vi "AWG Stop Pulses.vi"(8 "error in (no error)":errorcluster, 11 "awg session in":T1) -> (0 "error out":errorcluster, 3 "awg session out":T1)   [LabVIEW 2013, in "AWG.lvlib"]
doc: "AWG wrapper: Stops generation of pulses at output. At least for 33120 model this should be called first after initialization to stop standard waveform mode, i.e. to stop output."
uses:
  AWG.lvlib
  AWG Session.ctl
  AWG Type.ctl
  Agilent 33XXX Series/Agilent 33XXX Series.lvlib
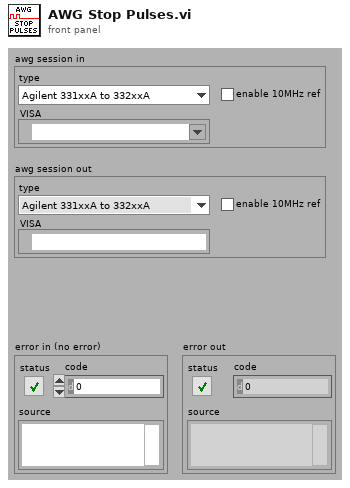
[diagram p1: front panel]
types:
  T1 = typedef "AWG.lvlib/AWG Session.ctl" = cluster{"type":T2, "VISA":refnum<visa-resource-name>, "enable 10MHz ref":bool}
  T2 = typedef "AWG.lvlib/AWG Type.ctl" = enum16{"Agilent 331xxA to 332xxA", "Agilent 335xxA to 336xxA", "dummy"}
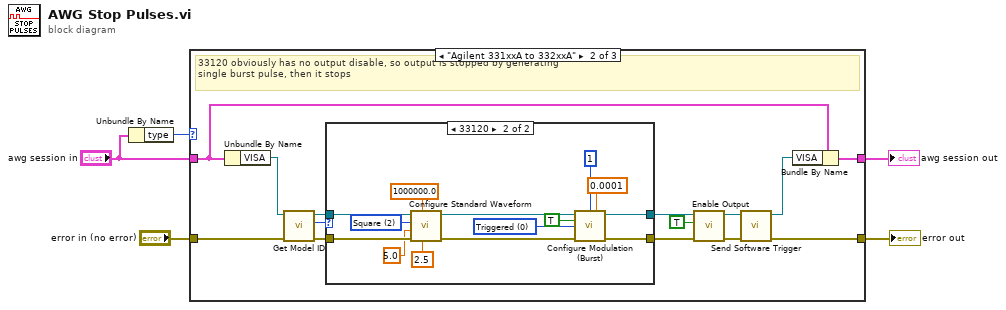
[diagram p0: block diagram]
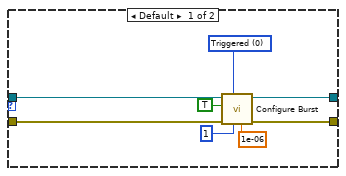
[diagram p3: hidden frame]
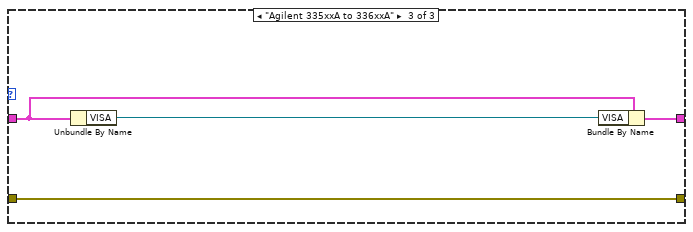
[diagram p4: hidden frame]
diagram:
  n1 = Unbundle By Name("awg session in") -> ("type"=w5:T2)
  n2 = case shown="\"Agilent 331xxA to 332xxA\"" w5 {
    tunnel: "error in (no error)" -> [w7 w19 w45]
    tunnel: [w7 w8 w45] -> w3
    tunnel: "awg session in" -> [w6 w20 w47]
    tunnel: [w6 w21 w46] -> w1
    frame Default {
    }
    frame "Agilent 331xxA to 332xxA" {
      # "33120 obviously has no output disable, so output is stopped by generating\nsingle burst pulse, then it stops"
      n3 = Unbundle By Name(w20) -> ("VISA"=w18:refnum<visa-resource-name>)
      n4 = call "Get Model ID.vi"("error in (no error)"=w19, "VISA resource name"=w18) -> ("error out"=w17:errorcluster, "model ID"=w15:u32, "VISA resource name out"=w16:refnum<visa-resource-name>)  [unwired: 7 in]
      n5 = case shown="33120" w15 {
        tunnel: [w23 w39] -> w13
        tunnel: [w22 w38] -> w12
        tunnel: w17 -> [w29 w37]
        tunnel: w16 -> [w28 w36]
        frame Default {
          w27 = u16 0 items=["Triggered", "Gated"] ("Burst Mode (0: Triggered)")
          n6 = call "Configure Burst.vi"("Burst Period (1 s)"=1e-06, "Burst Count (1)"=1, "Burst Mode (0: Triggered)"=w27, "error in (no error)"=w29, "Enable Burst (T: Enable)"=TRUE, "VISA resource name"=w28) -> ("error out"=w23:errorcluster, "VISA resource name out"=w22:refnum<visa-resource-name>)  [unwired: 4 in]
        }
        frame 33120 {
          w32 = u16 2 items=["DC", "Sine", "Square", "Triangle", "Ramp", "Pulse", "Noise", "Sinc", "Negative Ramp", "Exponential Rise", "Exponential Fall", "Cardiac"] ("Waveform Function (1: Sine)")
          w40 = u16 0 items=["Triggered", "Gated"] ("Burst Modulation Mode (0: Triggered)")
          n7 = call "Configure Standard Waveform.vi"("DC Offset (0.00 V)"=2.5, "Frequency (1000 Hz)"=1000000.0, "error in (no error)"=w37, "Amplitude (1)"=5.0, "Waveform Function (1: Sine)"=w32, "VISA resource name"=w36) -> ("error out"=w35:errorcluster, "VISA resource name out"=w34:refnum<visa-resource-name>)  [unwired: 4 in]
          n8 = call "Configure Modulation (Burst).vi"("VISA resource name"=w34, "Burst Count (1)"=1, "Burst Period (1 s)"=0.0001, "Enable Burst Modulation (T: Enable)"=TRUE, "Burst Modulation Mode (0: Triggered)"=w40, "error in (no error)"=w35) -> ("VISA resource name out"=w38:refnum<visa-resource-name>, "error out"=w39:errorcluster)  [unwired: 8 in]
        }
      }
      n9 = call "Enable Output.vi"("error in (no error)"=w13, "Enable Output  (T: Enable)"=TRUE, "VISA resource name"=w12) -> ("error out"=w11:errorcluster, "VISA resource name out"=w10:refnum<visa-resource-name>)  [unwired: 7 in]
      n10 = call "Send Software Trigger.vi"("error in (no error)"=w11, "VISA resource name"=w10) -> ("error out"=w8:errorcluster, "VISA resource name out"=w9:refnum<visa-resource-name>)  [unwired: 8 in]
      n11 = Bundle By Name(cluster=w20, "VISA"=w9) -> (w21:T1)
    }
    frame "Agilent 335xxA to 336xxA" {
      n12 = Unbundle By Name(w47) -> ("VISA"=w44:refnum<visa-resource-name>)
      n13 = Bundle By Name(cluster=w47, "VISA"=w44) -> (w46:T1)
    }
  }
  "error out" <- w3
  "awg session out" <- w1
